vi "Lab2_MainVI.vi"() -> ()   [LabVIEW 2020]
uses:
  <vilib>/MakerHub/LINX/Public/Utilities/Open Serial.vi
  <vilib>/addons/control/pid/pid.llb/PID (DBL).vi
  <vilib>/MakerHub/LINX/LMH-LINX.lvlib
  <vilib>/addons/control/pid/NI_PID_pid.lvlib
panel:
  out "Waveform Chart":cluster{dbl, "Setpoint":dbl}(graph)
  out "Hall Effect Voltage":dbl
  in  "Stop":bool
  in  "PWM Channel":u8
  in  "AI1 and AI2 Channels":u8[](array[numeric])
  in  "PID gains":T1={"proportional gain (Kc)"=1.0, "integral time (Ti, min)"=0.01, "derivative time (Td, min)"=0.0} {"derivative time (Td, min)" format="%.4f"; "integral time (Ti, min)" format="%.5f"; "proportional gain (Kc)" format="%.4f"}
  out "Duty Cycle":dbl format="%.2f"
  in  "Hall Analog Channel":u8
  in  "Serial Port":refnum<visa-resource-name>="N/A"
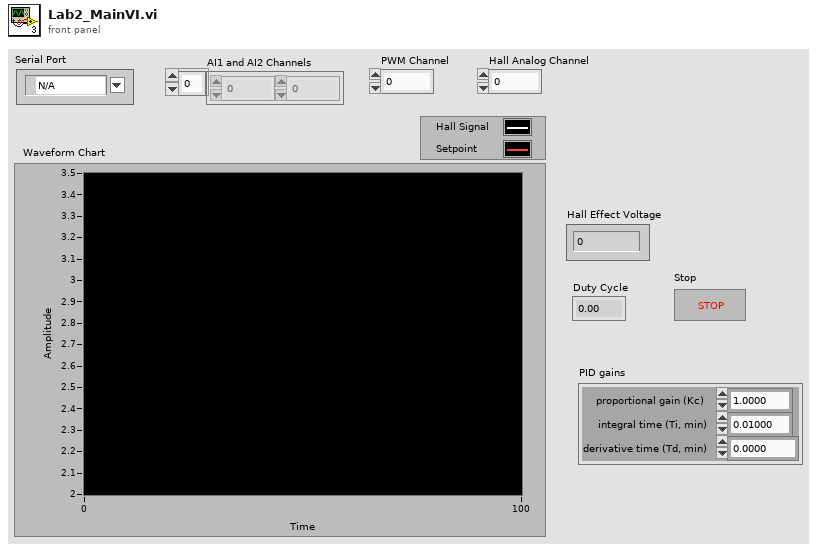
[diagram p1: front panel]
types:
  T1 = cluster{"proportional gain (Kc)":dbl, "integral time (Ti, min)":dbl, "derivative time (Td, min)":dbl}
  T2 = typedef "LMH-LINX.lvlib/LINX Ref.ctl" = cluster{"IO":T3, "Interface":T4, "LINX Device Config":T5}
  T3 = typedef "LMH-LINX.lvlib/Platform.ctl" = enum16{"Remote", "Local"}
  T4 = typedef "LMH-LINX.lvlib/Interface.ctl" = enum16{"Serial", "TCP"}
  T5 = typedef "LMH-LINX.lvlib/Device.lvlib/LINX Device Config.ctl" = cluster{"Interface":T4, "COM Port":refnum<visa-resource-name>, "TCP Configuration":T6, "Device Family":u8, "Device ID":u8, "Device Name":string, "TCP Ref":refnum<k5>, "Channels":T7}
  T6 = typedef "LMH-LINX.lvlib/Device.lvlib/TCP Config.ctl" = cluster{"IP Address":string, "Port":u16}
  T7 = typedef "LMH-LINX.lvlib/Channels.ctl" = cluster{"DI":u8[], "DO":u8[], "AI":u8[], "AO":u8[], "PWM":u8[], "QE":u8[], "UART":u8[], "I2C 2":u8[], "SPI":u8[], "CAN":u8[], "Servo":u8[], "AI Ref (V)":dbl, "AI Resolution (Bits)":u8, "AO Ref (V)":dbl, "AO Resolution (Bits)":u8}
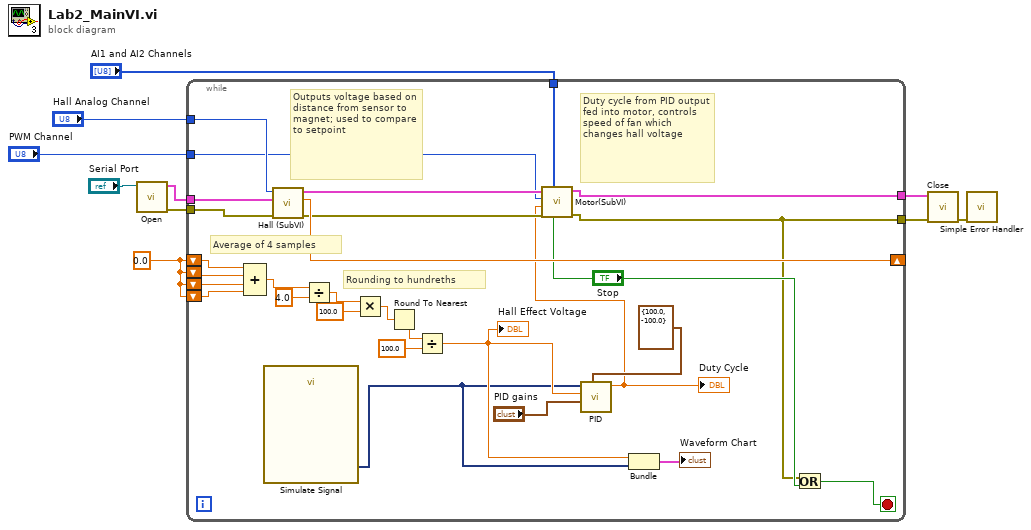
[diagram p0: block diagram]
diagram:
  w6 = 0.0 ("Hall Effect Voltage")
  n1 = call-poly <vilib>:"Open.vi"("Serial Port"="Serial Port") -> ("Error Out"=w7:errorcluster, "LINX Resource"=w9:T2)  [unwired: 8 in, 1 out]
  n2 = while {
    tunnel: w9 -> [w39]
    tunnel: "Hall Analog Channel" -> [w38]
    tunnel: w7 -> [w37]
    shift-right: [w36] -> _
    shift-left: w6 -> [w35]
    shift-left: w6 -> [w34]
    shift-left: w6 -> [w33]
    shift-left: w6 -> [w32]
    tunnel: "AI1 and AI2 Channels" -> [w21]
    tunnel: [w20] -> w4
    tunnel: "PWM Channel" -> [w19]
    tunnel: [w14] -> w2
    stop <- w16 stop-if-true
    # "Outputs voltage based on distance from sensor to magnet; used to compare to setpoint"
    # "Duty cycle from PID output fed into motor, controls speed of fan which changes hall voltage"
    # "Rounding to hundreths"
    # "Average of 4 samples"
    n3 = Compound Arithmetic op=ADD(w35, w34, w33, w32) -> (w31:dbl)
    n4 = call "Simulate Signal"() -> ("Sine"=w11:dynamicdata)  [unwired: 14 in, 1 out]
    n5 = call "Hall (SubVI).vi"("error in (no error)"=w37, "LINX  Input Resource"=w39, "Hall Analog Channel"=w38) -> ("error out"=w18:errorcluster, "Hall Effect Voltage"=w36:dbl, "LINX Output Resource"=w22:T2)  [unwired: 4 in, 2 out]
    n6 = Divide(x=w31, y=4.0) -> (x/y=w29:dbl)
    n7 = Multiply(x=w29, y=100.0) -> (x*y=w27:dbl)
    n8 = Round To Nearest(number=w27) -> (nearest integer value=w26:dbl)
    n9 = Divide(x=w26, y=100.0) -> (x/y=w13:dbl)
    "Hall Effect Voltage" <- w13
    n10 = call-poly <vilib>:"PID.vi"("output range"=cluster{"output high":dbl, "output low":dbl} {"output high"=100.0, "output low"=-100.0}, "PID gains"="PID gains", "process variable"=w13, "setpoint"=w11) -> ("output"=w17:dbl)  [unwired: 6 in, 1 out]
    "Duty Cycle" <- w17
    n11 = call "Motor(SubVI).vi"("Stop"="Stop", "AI1 and AI2 Channels"=w21, "error in (no error)"=w18, "Duty Cycle (-100 to +100)"=w17, "PWM Channel"=w19, "LINX  Input Resource"=w22) -> ("error out"=w14:errorcluster, "LINX Output Resource"=w20:T2)  [unwired: 3 in, 1 out]
    n12 = Bundle(w13, "Sine"=w11) -> (→"Waveform Chart":cluster{dbl, "Sine":dynamicdata})  [unwired: 1 in]
    n13 = Or(x=w14, y="Stop") -> (x .or. y?=w16:bool)
  }
  n14 = call <vilib>:"Close.vi"("Error In"=w2, "LINX Resource"=w4) -> ("Error Out"=w1:errorcluster)  [unwired: 9 in]
  n15 = call <vilib>:"Simple Error Handler.vi"("error in (no error)"=w1) -> ()  [unwired: 4 in, 5 out]
